vi "return_axis.vi"(7 "u(0)":sgl format="%#_13g", 8 "TsTicks":u32=1600, 11 "FPGA I/O In":refnum<k21>="Mod1/AO0") -> ()   [LabVIEW 2017]
uses:
  <vilib>/rvi/Emulation/niFpgaGetClockAttributes.vi
  <vilib>/rvi/Emulation/niFpgaSctlEmulationGetInTimedLoop.vi
  <vilib>/rvi/Emulation/niFpgaEmulationReportErrorSimple.vi
  <vilib>/rvi/eio/common/nirviEmuTemplateMethod_errors.vi
  <vilib>/rvi/Emulation/niFpgaCriticalErrorInLSC.vi
  <vilib>/eio/EIONode/EIONode.xnode
panel:
  out "Ux":sgl
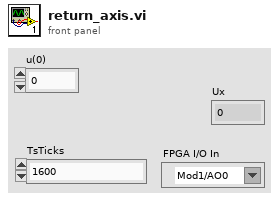
[diagram p1: front panel]
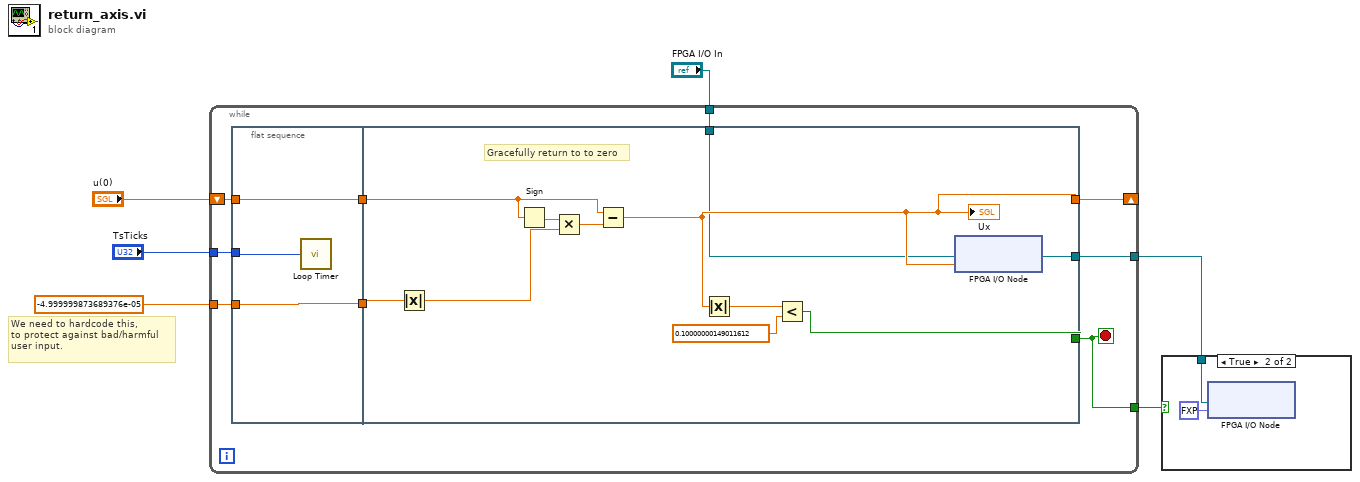
[diagram p0: block diagram]
diagram:
  # "We need to hardcode this,\nto protect against bad/harmful\nuser input."
  n1 = while {
    tunnel: sgl -5e-05 -> [w13]
    shift-right: [w12] -> _
    shift-left: "u(0)" -> [w11]
    tunnel: [w10] -> w5
    tunnel: "TsTicks" -> [w9]
    tunnel: "FPGA I/O In" -> [w8]
    tunnel: [w7] -> w1
    stop <- w10 stop-if-true
    n2 = flat-sequence {
      tunnel: [w18] -> w15
      tunnel: w11 -> [w18]
      tunnel: [w17] -> w14
      tunnel: w13 -> [w17]
      tunnel: w9 -> [w16]
      tunnel: w15 -> [w26]
      tunnel: w14 -> [w24]
      tunnel: [w21] -> w10
      tunnel: [w25] -> w12
      tunnel: w8 -> [w20]
      tunnel: [w19] -> w7
      frame #0 {
        n3 = call "Loop Timer"("Count(Ticks)"=w16) -> ()  [unwired: 1 out]
      }
      frame #1 {
        # "Gracefully return to to zero"
        n4 = Absolute Value(x=w24) -> (abs(x)=w23:sgl)
        n5 = Sign(1:w26) -> (0:w28:sgl)
        n6 = Multiply(x=w28, y=w23) -> (x*y=w29:sgl)
        n7 = Subtract(x=w26, y=w29) -> (x-y=w25:sgl)
        "Ux" <- w25
        n8 = Absolute Value(x=w25) -> (abs(x)=w27:sgl)
        n9 = Less?(x=w27, y=sgl 0.1) -> (x < y?=w21:bool)
        n10 = xnode "FPGA I/O Node"("I/O Item"=w25, "FPGA I/O In"=w20) -> ("FPGA I/O Out"=w19:refnum<k21>)
      }
    }
  }
  n11 = case shown="True" w5 {
    tunnel: w1 -> [_ w31]
    frame False {
    }
    frame True {
      n12 = xnode "FPGA I/O Node"("I/O Item"=fxp<+/-,20,5> 0.0, "FPGA I/O In"=w31) -> ()  [unwired: 1 out]
    }
  }
